vi "QC_RunInformation.vi"() -> ()   [LabVIEW 2018]
panel:
  out "LocalConfiguration":T1={"Institute"="FZU", "Manufacturers"=["Hamamatsu"], "Devices"=["ATLAS07", "ATLAS12", "ATLAS12EC", "ATLAS17LS", "ATLAS18SS", "ATLAS18R0", "ATLAS18R1", "ATLAS18R2", "ATLAS18R3", "ATLAS18R4", "ATLAS18R5", "HALFMOON"], "Serialnumbers Lookup DB"="C:\\Users\\veral\\Documents\\christoph\\LabVIEW 2013\\general_VIs\\database\\components.csv", "Data directory"="C:\\Users\\veral\\Documents\\cambridge-data-test\\data", "Backup & screenshot directory"="C:\\Users\\veral\\Documents\\cambridge-data-test\\backup", "List of known users"=["Vera", "Marcela", "Iveta"], "Measurement switch not used"=TRUE, "Measurement Switch"="Pickering Matrix", "DUT Switch"="Keithley 3706A", "Rseries IV [MOhm]"="1.0", "Rshunt IV [MOhm]"="0.00", "Rseries CV [MOhm]"="1.0", "DC blocking Cap [µF]"="2.2", "Rseries LCR [MOhm]"="1.0", "Rseries stability [MOhm]"="13.2", "Rshunt stability [MOhm]"="1.0", "Rseries striptest bias [MOhm]"="0.1", "Rseries strip pinhole [MOhm]"="2.2"}
  in  "Run info":T2={"Sensor Serial No.:"="2", "Wafer:"="2", "Batch:"="3", "Manufacturer:"="Hamamatsu", "Device Category:"="ATLAS07", "Database Serial No.:"="1", "Date Initiated:"="23 Sep 2020", "Time Initiated:"="14:51:49", "Test"="SENSOR_IV", "Probeplan used:"="", "End of Run comment:"="Run aborted - by user", "User:"="Vera", "Vbias SMU"="", "LCR"="", "Test SMU"="", "Test DMM"=""}
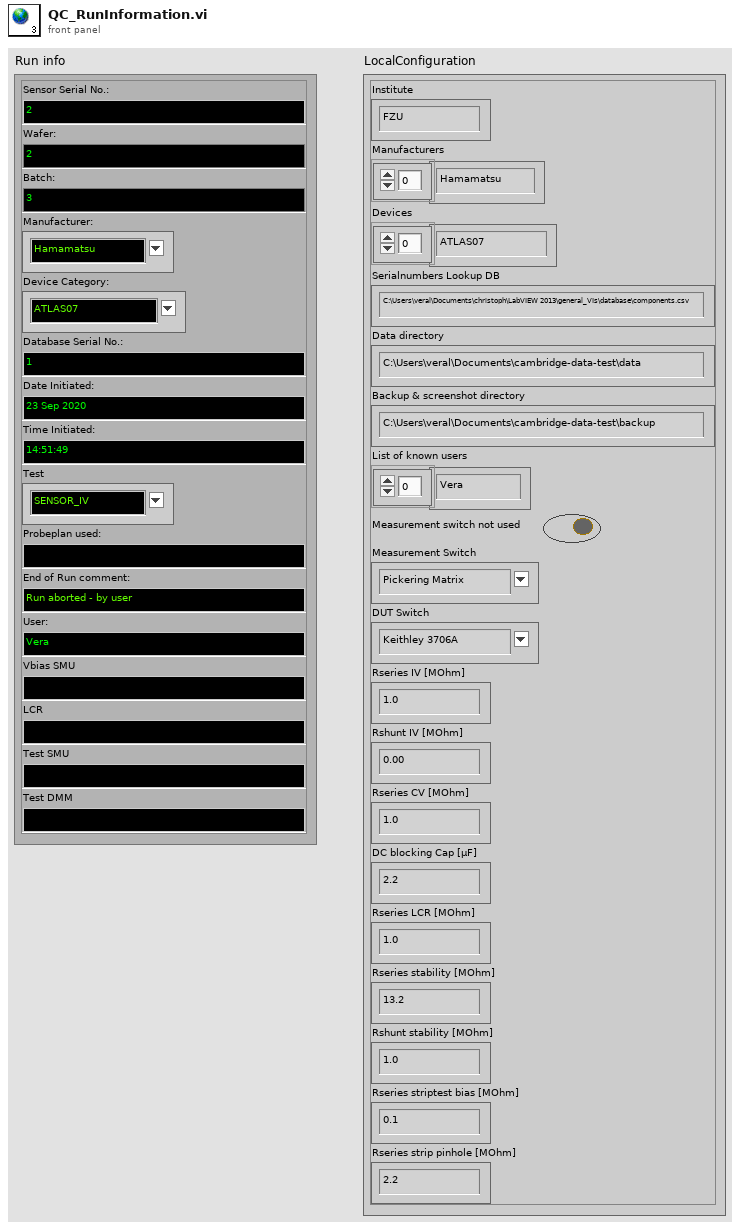
[diagram p1: front panel]
types:
  T1 = cluster{"Institute":string, "Manufacturers":string[], "Devices":string[], "Serialnumbers Lookup DB":string, "Data directory":string, "Backup & screenshot directory":string, "List of known users":string[], "Measurement switch not used":bool, "Measurement Switch":string, "DUT Switch":string, "Rseries IV [MOhm]":string, "Rshunt IV [MOhm]":string, "Rseries CV [MOhm]":string, "DC blocking Cap [µF]":string, "Rseries LCR [MOhm]":string, "Rseries stability [MOhm]":string, "Rshunt stability [MOhm]":string, "Rseries striptest bias [MOhm]":string, "Rseries strip pinhole [MOhm]":string}
  T2 = cluster{"Sensor Serial No.:":string, "Wafer:":string, "Batch:":string, "Manufacturer:":string, "Device Category:":string, "Database Serial No.:":string, "Date Initiated:":string, "Time Initiated:":string, "Test":string, "Probeplan used:":string, "End of Run comment:":string, "User:":string, "Vbias SMU":string, "LCR":string, "Test SMU":string, "Test DMM":string}
diagram:
